vi "ToRepo.vi"(8 "error in":errorcluster, 9 "to repo cluster":T1, 10 "repository in":refnum<class "NISE_CEF_Repository.lvclass">, 11 "channel in":refnum<class "Channel.lvclass">) -> (0 "error out":errorcluster, 2 "repository out":refnum<class "NISE_CEF_Repository.lvclass">, 3 "channel out":refnum<class "Channel.lvclass">)   [LabVIEW 2013, in "Channel.lvclass"]
uses:
  Channel.lvclass
  Configuration Framework/Repository/NISE_CEF_Repository.lvclass
  Configuration Framework/Node/ToRepoCluster.ctl
  cRIO Repo/cRIORepo.lvclass
  Channel.lvclass/Channel.ctl
  Configuration Framework/Node/NISE_CEF_Node.lvclass
  cRIO Repo/cRIORepo.lvclass/cRIORepo.ctl
  Read Channel info.vi
  cRIO Repo/Read Channels.vi
  cRIO Repo/Read Channel Group.vi
  cRIO Repo/Read System.vi
  cRIO Repo/Write Channels.vi
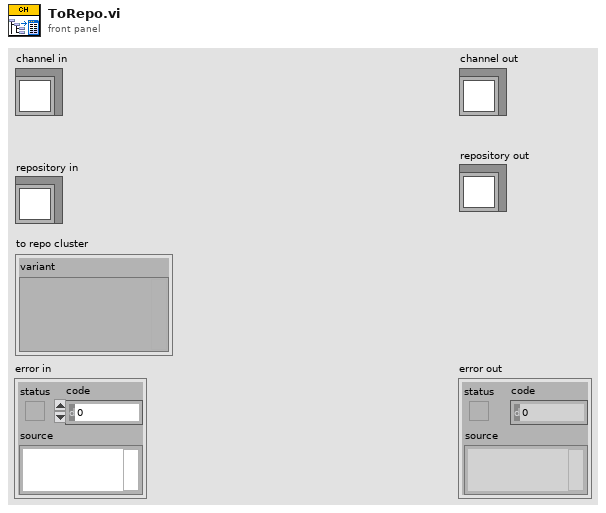
[diagram p1: front panel]
types:
  T1 = typedef "NISE_CEF_Node.lvclass/ToRepoCluster.ctl" = cluster{"variant":variant}
  T2 = typedef "Channel.ctl" = cluster{"channel group":string, "channel name":string, "IO ":string, "sensor ID":string, "description":string, "system":string, "channel type":string}
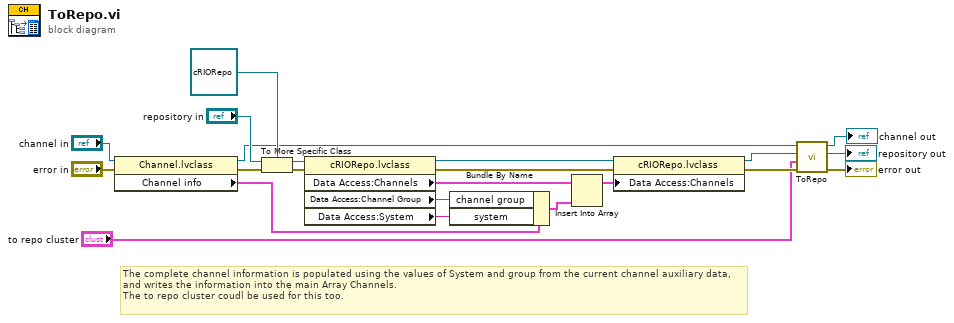
[diagram p0: block diagram]
diagram:
  # "The complete channel information is populated using the values of System and group from the current channel auxiliary data, and writes the information into the main Array Channels.\nThe to repo cluster coudl be used for this too."
  n1 = property class="Channel.lvclass"(reference="channel in", error in="error in") -> (reference out=w13:refnum<class "Channel.lvclass">, error out=w15:errorcluster, "Channel info"=w2:T2)
  n2 = To More Specific Class(target class=refnum<class "cRIORepo.lvclass"> refnum ("cRIO repo.lvclass"), reference="repository in", error in=w15) -> (specific class reference=w18:refnum<class "cRIORepo.lvclass">, error out=w14:errorcluster)
  n3 = property class="cRIORepo.lvclass"(reference=w18, error in=w14) -> (reference out=w9:refnum<class "cRIORepo.lvclass">, error out=w10:errorcluster, "Data Access:Channels"=w8:T2[], "Data Access:Channel Group"=w4:string, "Data Access:System"=w3:string)
  n4 = Bundle By Name(cluster=w2, "channel group"=w4, "system"=w3) -> (w7:T2)
  n5 = Insert Into Array(array=w8, new element=w7) -> (w6:T2[])  [unwired: 1 in]
  n6 = property class="cRIORepo.lvclass"(reference=w9, error in=w10, "Data Access:Channels"=w6) -> (reference out=w5:refnum<class "cRIORepo.lvclass">, error out=w11:errorcluster)
  n7 = call-parent "ToRepo.vi"("error in"=w11, "to repo cluster"="to repo cluster", "repository in"=w5, "node in"=w13) -> ("error out"=→"error out":errorcluster, "repository out"=→"repository out":refnum<class "NISE_CEF_Repository.lvclass">, "node out"=→"channel out":refnum<class "Channel.lvclass">)  [unwired: 5 in]
